vi "Max Search.vi"() -> ()   [LabVIEW 2024]
panel:
  out "Max":dbl
  out "Random Number":dbl
  out "Iteration Count":i32
  in  "Number of Iterations":i32
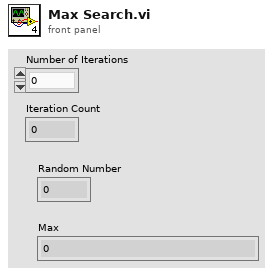
[diagram p1: front panel]
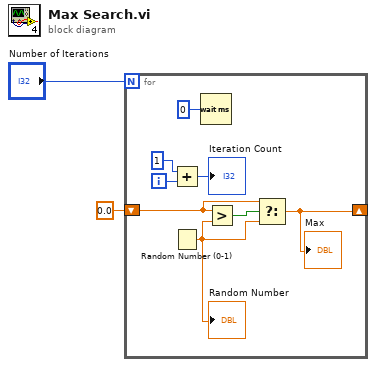
[diagram p0: block diagram]
diagram:
  n1 = for {
    N: "Number of Iterations" -> [_]
    shift-right: [w3] -> _
    shift-left: 0.0 -> [w4]
    i -> [w8]
    n2 = Add(x=1, y=w8) -> (x+y=→"Iteration Count":i32)
    n3 = Random Number (0-1)() -> (number: 0 to 1=w6:dbl)
    "Random Number" <- w6
    n4 = Wait (ms)(milliseconds to wait=u32 0) -> ()  [unwired: 1 out]
    n5 = Greater?(x=w4, y=w6) -> (0:w7:bool)
    n6 = Select(t=w4, s=w7, f=w6) -> (s? t:f=w3:dbl)
    "Max" <- w3
  }
